vi "Maui.Config.Create.vi"(8 "error in (no error)":errorcluster, 10 "Owning Class":refnum<class>, 11 "Maui.Config in":refnum<class "Maui.Config.lvclass">) -> (0 "error out":errorcluster, 3 "Maui.Config out":refnum<class "Maui.Config.lvclass">)   [LabVIEW 2019, in "Maui.Config.lvclass"]
uses:
  Maui.Config.lvclass
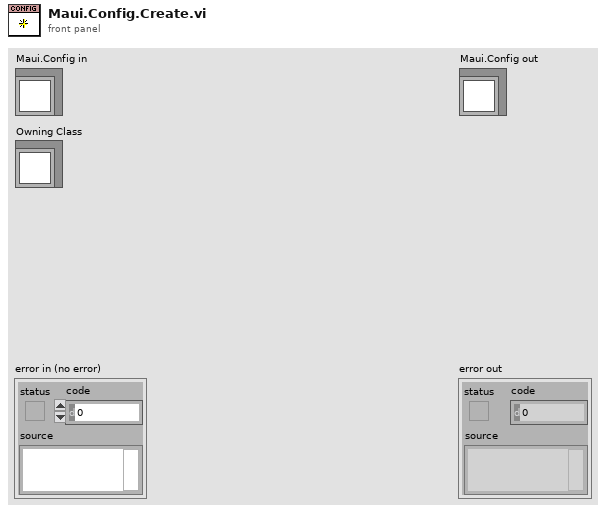
[diagram p1: front panel]
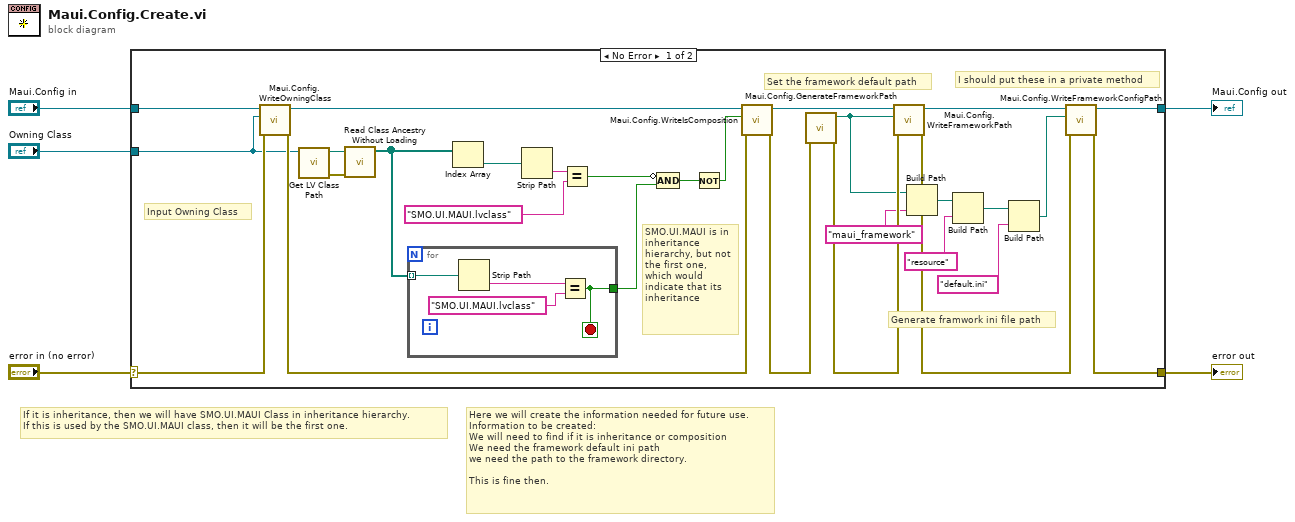
[diagram p0: block diagram]
diagram:
  # "Here we will create the information needed for future use.\nInformation to be created:\nWe will need to find if it is inheritance or composition\nWe need the framework default ini path\nwe need the path to the framework directory.\n\nThis is fine then."
  # "If it is inheritance, then we will have SMO.UI.MAUI Class in inheritance hierarchy.\nIf this is used by the SMO.UI.MAUI class, then it will be the first one."
  n1 = case shown="No Error" "error in (no error)" {
    selector: "error in (no error)" -> [w33 w40]
    tunnel: [w9 w40] -> w4
    tunnel: [w15 w39] -> w2
    tunnel: "Maui.Config in" -> [w34 w39]
    tunnel: "Owning Class" -> [w25 _]
    frame No Error {
      # "I should put these in a private method"
      # "Generate framwork ini file path"
      # "SMO.UI.MAUI is in inheritance hierarchy, but not the first one, which would indicate that its inheritance"
      # "Set the framework default path"
      # "Input Owning Class"
      n2 = call "Maui.Config.WriteOwningClass.vi"("error in (no error)"=w33, "Owning Class"=w25, "Maui.Config in"=w34) -> ("error out"=w31:errorcluster, "Maui.Config out"=w32:refnum<class "Maui.Config.lvclass">)  [unwired: 7 in]
      n3 = call <vilib>:"Get LV Class Path.vi"("object"=w25) -> ("error out"=w27:errorcluster, "class path"=w26:path)  [unwired: 9 in]
      n4 = call <vilib>:"Read Class Ancestry Without Loading.vi"("error in (no error)"=w27, "LabVIEW Class Path"=w26) -> ("Class Ancestry"=w24:path[])  [unwired: 8 in, 1 out]
      n5 = for {
        tunnel: [w35] -> w19
        tunnel: w24 -> [w36] mode=indexing
        stop <- w35 stop-if-true
        n6 = Strip Path(path=w36) -> (name=w38:string)  [unwired: 1 out]
        n7 = Equal?(x=w38, y="SMO.UI.MAUI.lvclass") -> (x = y?=w35:bool)
      }
      n8 = Index Array(array=w24) -> (element=w23:path)  [unwired: 1 in]
      n9 = Strip Path(path=w23) -> (name=w22:string)  [unwired: 1 out]
      n10 = Equal?(x=w22, y="SMO.UI.MAUI.lvclass") -> (x = y?=w20:bool)
      n11 = Compound Arithmetic op=AND(invert w20, w19) -> (w18:bool)
      n12 = Not(x=w18) -> (.not. x?=w17:bool)
      n13 = call "Maui.Config.WriteIsComposition.vi"("error in (no error)"=w31, "Composition"=w17, "Maui.Config in"=w32) -> ("error out"=w29:errorcluster, "Maui.Config out"=w30:refnum<class "Maui.Config.lvclass">)  [unwired: 7 in]
      n14 = call "Maui.Config.GenerateFrameworkPath.vi"("error in (no error)"=w29) -> ("error out"=w28:errorcluster, "Framework Path"=w8:path)  [unwired: 8 in, 1 out]
      n15 = call "Maui.Config.WriteFrameworkPath.vi"("error in (no error)"=w28, "Framework Path"=w8, "Maui.Config in"=w30) -> ("error out"=w7:errorcluster, "Maui.Config out"=w16:refnum<class "Maui.Config.lvclass">)  [unwired: 7 in]
      n16 = Build Path(base path=w8, name or relative path="maui_framework") -> (appended path=w13:path)
      n17 = Build Path(base path=w13, name or relative path="resource") -> (appended path=w11:path)
      n18 = Build Path(base path=w11, name or relative path="default.ini") -> (appended path=w6:path)
      n19 = call "Maui.Config.WriteFrameworkConfigPath.vi"("error in (no error)"=w7, "Framework Configuration"=w6, "Maui.Config in"=w16) -> ("error out"=w9:errorcluster, "Maui.Config out"=w15:refnum<class "Maui.Config.lvclass">)  [unwired: 7 in]
    }
    frame Error {
    }
  }
  "error out" <- w4
  "Maui.Config out" <- w2
